vi "DSF.Engine.Memory.BufferPool.Deallocate.vi"(8 "error in (no error)":errorcluster, 11 "BufferPool":refnum<class "DSF.Engine.Memory.BufferPool.lvclass">) -> (0 "error out":errorcluster)   [LabVIEW 2016, in "DSF.Engine.lvlib" / "DSF.Engine.Memory.BufferPool.lvclass"]
uses:
  BufferPool/DSF.Engine.Memory.BufferPool.lvclass
  BufferPool/DSF.Engine.Memory.BufferPool.lvclass/DSF.Engine.Memory.BufferPool.ctl
  Buffer/DSF.Engine.Memory.Buffer.lvclass
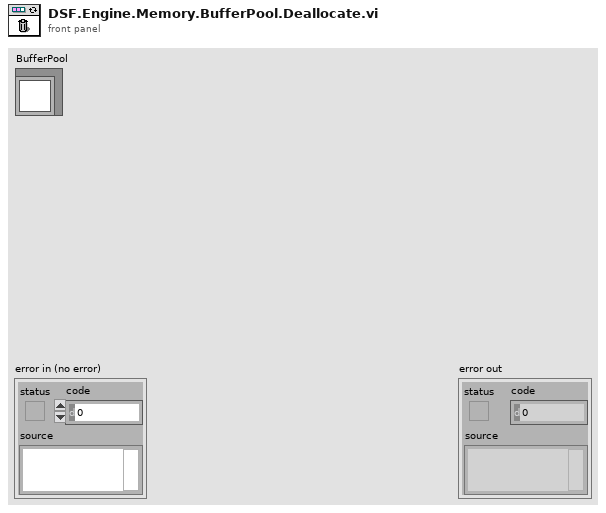
[diagram p1: front panel]
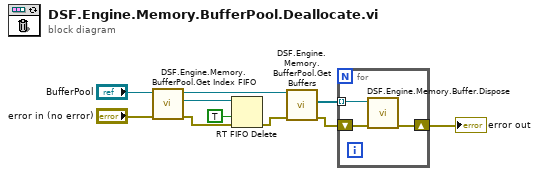
[diagram p0: block diagram]
diagram:
  n1 = call "DSF.Engine.Memory.BufferPool.Get Index FIFO.vi"("error in (no error)"="error in (no error)", "BufferPool in"="BufferPool") -> ("error out"=w4:errorcluster, "Index FIFO"=w8:refnum<k33>, "BufferPool out"=w6:refnum<class "DSF.Engine.Memory.BufferPool.lvclass">)  [unwired: 7 in]
  n2 = RT FIFO Delete(0:w8, 2:TRUE ("force destroy? (F)"), 3:w4) -> (11:w7:errorcluster)
  n3 = call "DSF.Engine.Memory.BufferPool.Get Buffers.vi"("error in (no error)"=w7, "BufferPool in"=w6) -> ("error out"=w2:errorcluster, "Buffers"=w1:refnum<class "DSF.Engine.Memory.Buffer.lvclass">[])  [unwired: 7 in, 1 out]
  n4 = for {
    shift-right: [w11] -> w3
    shift-left: w2 -> [w13]
    tunnel: w1 -> [w12] mode=indexing
    n5 = call "DSF.Engine.Memory.Buffer.Dispose.vi"("error in (no error)"=w13, "Buffer in"=w12) -> ("error out"=w11:errorcluster)  [unwired: 9 in]
  }
  "error out" <- w3
